vi "Destroy.vi"   [LabVIEW 2018, in "Toolkit.lvlib" / "Listener.lvclass"]
uses:
  Listener.lvclass
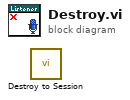
[diagram p0: block diagram]
diagram:
  n1 = call "Destroy to Session.vi"() -> ()  [unwired: 10 in, 2 out]
